vi "Quit Application.vi"(8 "error in (no error)":errorcluster, 10 "window name (\"\")":string, 11 "window refnum (NaWR)":T1) -> (0 "error out":errorcluster)   [LabVIEW 2023, in "Winevent.lvlib"]
doc: "This VI will close the application identified by window ID in or by the name of the application window. Note that the window to be closed must have no owner or parent window.\n\nFor example, this VI will not work if sent to another LabVIEW VI window - use LabVIEW's built-in Exit function to quit LabVIEW."
uses:
  WINUTIL/Window Refnum.ctl
  Winevent.lvlib
  WINUTIL/WINUTIL.lvlib
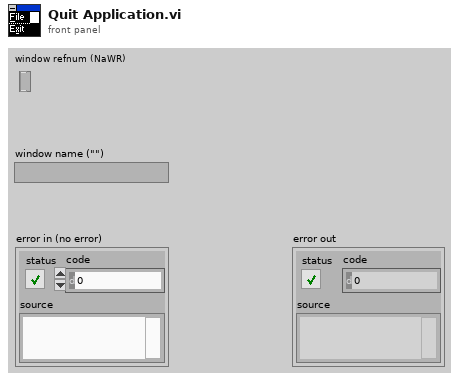
[diagram p1: front panel]
types:
  T1 = typedef "WINUTIL.lvlib/Window Refnum.ctl" = refnum<k1>
  T2 = enum8{"Maximize Window", "Minimize Window", "Show Task List", "Start Screen Saver", "Quit Application"}
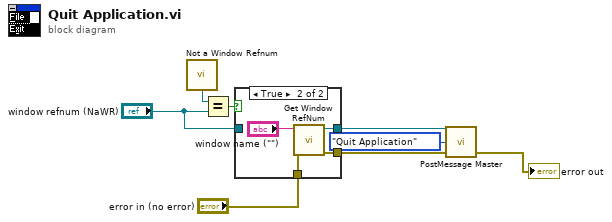
[diagram p0: block diagram]
diagram:
  n1 = call "Not a Window Refnum.vi"() -> ("Not a Window Refnum"=w2:T1)
  n2 = Equal?(x=w2, y="window refnum (NaWR)") -> (x = y?=w3:bool)
  n3 = case shown="True" w3 {
    tunnel: "error in (no error)" -> [w9 w13]
    tunnel: [w10 w12] -> w6
    tunnel: [w9 w11] -> w5
    tunnel: "window refnum (NaWR)" -> [w10 _]
    frame False {
    }
    frame True {
      n4 = call "Get Window RefNum.vi"("error in (no error)"=w13, "window name (\"\")"="window name (\"\")") -> ("error out"=w11:errorcluster, "window refnum (NaWR)"=w12:T1)  [unwired: 6 out]
    }
  }
  n5 = call "PostMessage Master.vi"("window refnum"=w6, "function"=T2."Quit Application", "error in (no error)"=w5) -> ("error out"=→"error out":errorcluster)  [unwired: 1 in, 3 out]
